vi "IsValidCoordinate.vi"(1 "Column":u32, 2 "Row":u32) -> (0 "Valid":bool)   [LabVIEW 2025]
uses:
  server/ServerGlobalVariables.vi
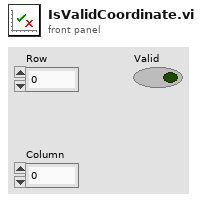
[diagram p1: front panel]
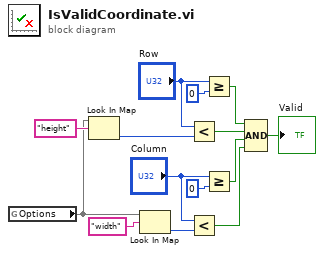
[diagram p0: block diagram]
diagram:
  n1 = global read "ServerGlobalVariables.vi" "Options"() -> (w1:map{string, u32})
  n2 = Look In Map(map=w1, key="height") -> (value=w6:u32)  [unwired: 1 in, 1 out]
  n3 = Look In Map(map=w1, key="width") -> (value=w8:u32)  [unwired: 1 in, 1 out]
  n4 = Less?(x="Row", y=w6) -> (x < y?=w12:bool)
  n5 = Less?(x="Column", y=w8) -> (x < y?=w10:bool)
  n6 = Greater Or Equal?(x="Row", y=u32 0) -> (x >= y?=w13:bool)
  n7 = Greater Or Equal?(x="Column", y=u32 0) -> (x >= y?=w11:bool)
  n8 = Compound Arithmetic op=AND(w13, w12, w11, w10) -> (→"Valid":bool)
